vi "GetStringArray.vi"(4 "Sequence Context":T1) -> (0 "error out":errorcluster, 1 "Test Data":T2 {"Numeric Measurement" format="%.2f"})   [LabVIEW 2011]
uses:
  <vilib>/addons/TestStand/_TSLegacy.llb/LabVIEW Test - Test Data.ctl
  <vilib>/addons/TestStand/_TSLegacy.llb/LabVIEW Test - Sequence Context.ctl
panel:
  in  "Boolean":bool
  out "Value":string[](array[string])
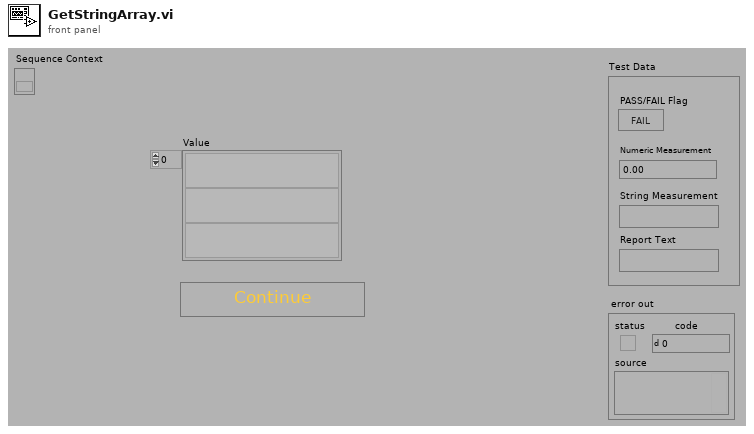
[diagram p1: front panel]
types:
  T1 = typedef "LabVIEW Test - Sequence Context.ctl" = refnum<k7>
  T2 = typedef "LabVIEW Test - Test Data.ctl" = cluster{"PASS/FAIL Flag":bool, "Numeric Measurement":dbl, "String Measurement":string, "Report Text":string}
  T3 = cluster{"Execution":refnum<k7>, "InitTerminationMonitor":refnum<k7>, "Sequence Context Out":refnum<k7>}
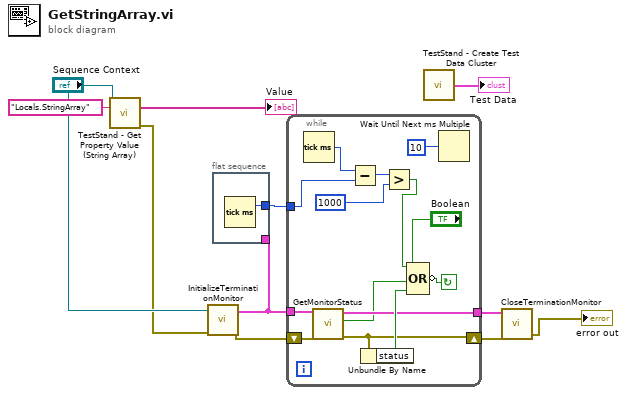
[diagram p0: block diagram]
diagram:
  n1 = call <vilib>:"TestStand - Get Property Value (String Array).vi"("Sequence Context In"="Sequence Context", "Lookup String"="Locals.StringArray") -> ("Value"=→"Value":string[], "error out"=w3:errorcluster)  [unwired: 1 in, 11 out]
  n2 = call <vilib>:"InitializeTerminationMonitor.vi"("error in (no error)"=w3, "Sequence Context In"="Sequence Context") -> ("error out"=w6:errorcluster, "StatusMonitor Out"=w2:T3)  [unwired: 8 out]
  n3 = flat-sequence {
    tunnel: [w12] -> w1
    tunnel: w2 -> [_]
    frame #0 {
      n4 = Tick Count (ms)() -> (millisecond timer value=w12:u32)
    }
  }
  n5 = while {
    tunnel: [w20] -> w4
    tunnel: w2 -> [w21]
    shift-left: w6 -> [w23]
    shift-right: [w22] -> w5
    tunnel: w1 -> [w14]
    stop <- w25 continue-if-true
    n6 = Tick Count (ms)() -> (millisecond timer value=w16:u32)
    n7 = call <vilib>:"GetMonitorStatus.vi"("error in"=w23, "StatusMonitor In"=w21) -> ("error out"=w22:errorcluster, "GetTerminationMonitorStatus"=w19:bool, "StatusMonitor Out"=w20:T3)  [unwired: 3 out]
    n8 = Subtract(x=w16, y=w14) -> (x-y=w15:u32)
    n9 = Unbundle By Name(w22) -> ("status"=w26:bool)
    n10 = Greater?(x=w15, y=u32 1000) -> (0:w13:bool)
    n11 = Compound Arithmetic op=OR(w13, "Boolean", w19, w26) -> (invert w25:bool)
    n12 = Wait Until Next ms Multiple(millisecond multiple=u32 10) -> ()  [unwired: 1 out]
  }
  n13 = call <vilib>:"TestStand - Create Test Data Cluster.vi"() -> ("Test Data"=→"Test Data":T2)  [unwired: 4 in]
  n14 = call <vilib>:"CloseTerminationMonitor.vi"("error in"=w5, "StatusMonitor In"=w4) -> ("error out"=→"error out":errorcluster)  [unwired: 3 out]
